vi "c_ctre_phoenix6_set_configs.vi"(0 "Numeric 2":i32, 1 "String 2":string, 2 "Numeric 3":i32, 3 "Numeric 4":dbl, 4 "String 4":string, 5 "Numeric 5":u32, 6 "Numeric 6":u8, 7 "Numeric 7":u8, 8 "Numeric 8":u8) -> (20 "Numeric":i32, 21 "String":string, 22 "String 3":string)   [LabVIEW 2023]
uses:
  <vilib>/Rock Robotics/WPI/ThirdParty/Phoenix-LabVIEW/Controls/DriverLib.ctl
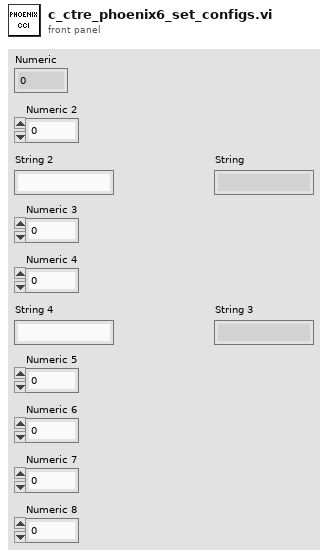
[diagram p1: front panel]
types:
  T1 = typedef "DriverLib.ctl" = path
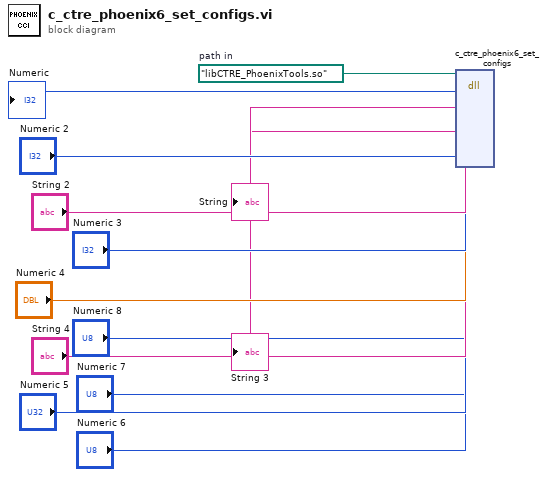
[diagram p0: block diagram]
diagram:
  w13 = T1 path "libCTRE_PhoenixTools.so"  # path in
  n1 = dll-call lib="?" fn="c_ctre_phoenix6_set_configs"(path in=w13, "Numeric 2", "String 2", "Numeric 3", "Numeric 4", "String 4", "Numeric 5", "Numeric 6", "Numeric 7", "Numeric 8") -> (→"Numeric":i32, →"String":string, →"String 3":string)  [unwired: 9 in, 2 out]
